vi "Add.vi"(10 "Right":refnum<class "SnailNum.lvclass">, 11 "Left":refnum<class "SnailNum.lvclass">) -> (3 "SnailNum":refnum<class "SnailNum.lvclass">)   [LabVIEW 2020]
uses:
  SnailNum.lvclass
  Set Left.vi
  Set Right.vi
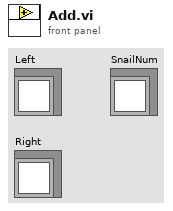
[diagram p1: front panel]
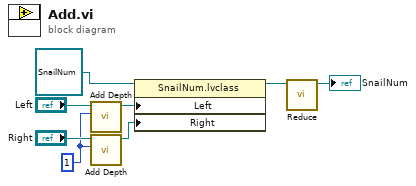
[diagram p0: block diagram]
diagram:
  w2 = 1 ("Delta Depth")
  n1 = call "Add Depth.vi"("Delta Depth"=w2, "SnailNum in"="Left") -> ("SnailNum out"=w5:refnum<class "SnailNum.lvclass">)  [unwired: 8 in, 1 out]
  n2 = call "Add Depth.vi"("Delta Depth"=w2, "SnailNum in"="Right") -> ("SnailNum out"=w3:refnum<class "SnailNum.lvclass">)  [unwired: 8 in, 1 out]
  n3 = property class="SnailNum.lvclass"(reference=refnum<class "SnailNum.lvclass"> refnum ("SnailNum.lvclass"), "Left"=w5, "Right"=w3) -> (reference out=w7:refnum<class "SnailNum.lvclass">)  [unwired: 1 in, 1 out]
  n4 = call "Reduce.vi"("SnailNum in"=w7) -> ("SnailNum out"=→"SnailNum":refnum<class "SnailNum.lvclass">)  [unwired: 9 in, 1 out]
